vi "CSV_AppendNewCol_UT.vi"   [LabVIEW 2015, in "LVdataToTableData.lvlib"]
uses:
  LVdataToTableData.lvlib
types:
  T1 = cluster{"Str":string, "Str1 (A, B, C, D)":string[], "Str2":string[]}
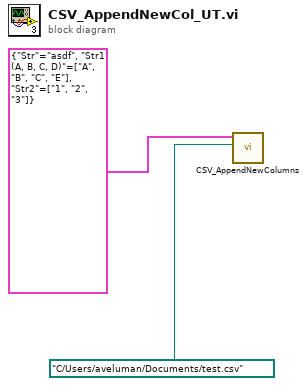
[diagram p0: block diagram]
diagram:
  n1 = call "CSV_AppendNewColumns.vi"("New/Existing CSV file path"=path "C:/Users/aveluman/Documents/test.csv" ("file path (dialog if empty)"), "New Data"=T1 {"Str"="asdf", "Str1 (A, B, C, D)"=["A", "B", "C", "E"], "Str2"=["1", "2", "3"]}) -> ()  [unwired: 7 in, 3 out]
